vi "_056.vi"() -> ()   [LabVIEW 2024]
panel:
  out "Random Data (Shift Register)":dbl[](graph)
  out "Random Data (Feedback Node)":dbl[](graph)
  in  "stop":bool
  # "Shift Register & FeedBack Node :"
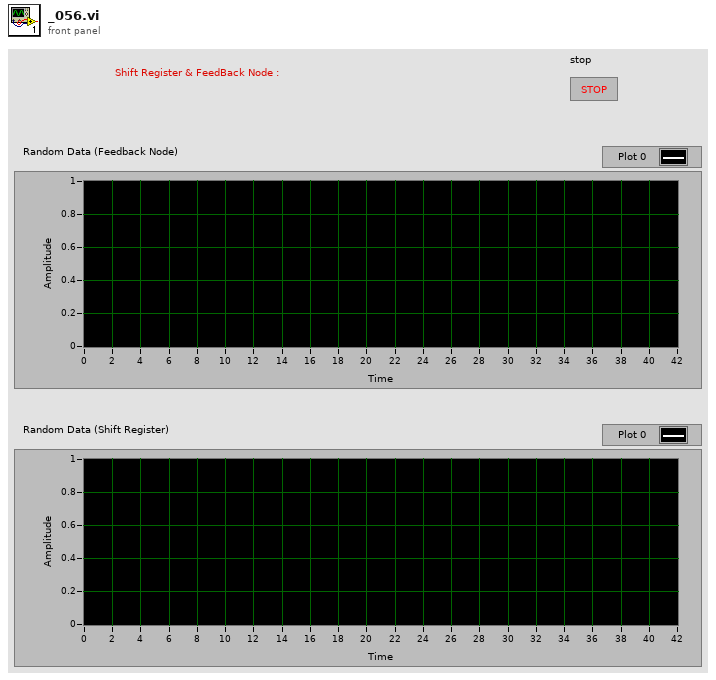
[diagram p1: front panel]
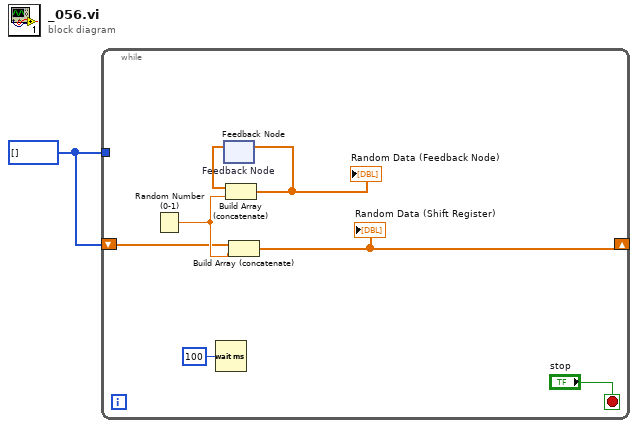
[diagram p0: block diagram]
diagram:
  w1 = i32[] []
  n1 = while {
    shift-right: [w2] -> _
    shift-left: w1 -> [w3]
    tunnel: w1 -> [_]
    stop <- "stop" stop-if-true
    n2 = Random Number (0-1)() -> (number: 0 to 1=w6:dbl)
    n3 = Wait (ms)(milliseconds to wait=u32 100) -> ()  [unwired: 1 out]
    n4 = feedback #1 "Feedback Node"() -> (w5:dbl[])  [unwired: 1 in]
    n5 = Build Array (concatenate)(w5, w6) -> (w4:dbl[])
    "Random Data (Feedback Node)" <- w4
    n6 = feedback-in #1(w4) -> ()
    n7 = Build Array (concatenate) "Build Array"(w3, w6) -> (w2:dbl[])
    "Random Data (Shift Register)" <- w2
  }
